vi "Write CPU Done.vi"(8 "error in (no error)":errorcluster, 10 "CPU Done":refnum<user-event>, 11 "Simple UI in":refnum<class "Simple UI.lvclass">) -> (0 "error out":errorcluster, 3 "Simple UI out":refnum<class "Simple UI.lvclass">)   [LabVIEW 2020, in "Simple UI.lvlib" / "Simple UI.lvclass"]
uses:
  Simple UI.lvclass
  Simple UI.lvclass/Simple UI.ctl
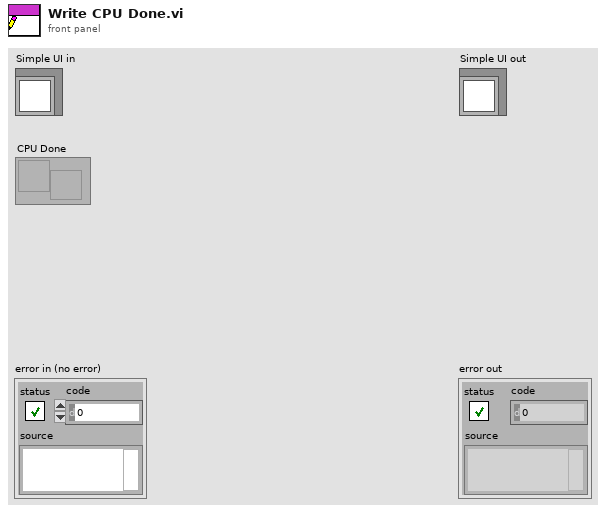
[diagram p1: front panel]
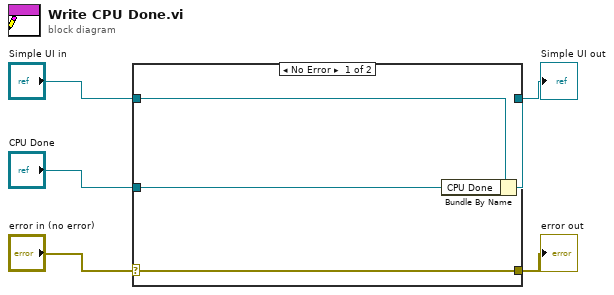
[diagram p0: block diagram]
diagram:
  n1 = case shown="No Error" "error in (no error)" {
    selector: "error in (no error)" -> [w9 w10]
    tunnel: [w9 w10] -> w4
    tunnel: [w7 w11] -> w2
    tunnel: "Simple UI in" -> [w8 w11]
    tunnel: "CPU Done" -> [w6 _]
    frame No Error {
      n2 = Bundle By Name(cluster=w8, "CPU Done"=w6) -> (w7:refnum<class "Simple UI.lvclass">)
    }
    frame Error {
    }
  }
  "error out" <- w4
  "Simple UI out" <- w2
